vi "oax_Check DAQ Config (DSA).vi"(8 "error in (no error)":errorcluster, 10 "Tacho Type":enum16{"Analog Tacho", "Digital Tacho"}(ring), 11 "DAQ Config":T1 {"pregain" format="%.2f"; "IEPE" items=["On", "Off", "None"]; "coupling" items=["DC", "AC"]; "engineering units" items=["custom..."=0, "V"=1, "A"=21, "C"=30, "pC"=31, "s"=32, "-"=29, "Pa"=2, "N"=20, "g"=3, "m/s^2"=4, "m/s"=5, "m"=6, "mm/s"=12, "mm"=13, "micron/s"=14, "micron"=15, "in/s^2"=7, "in/s"=8, "in"=9, "mil/s"=10, "mil"=11, "rad/s^2"=16, "rad/s"=17, "rad"=18, "deg/s^2"=26, "deg/s"=27, "deg"=28, "RPM"=22, "cycle/s^2"=23, "Hz"=24, "cycle"=25, "strain"=19]; "sensor sensitivity (mV/EU)" format="%.2f"; "dB reference" format="%.1e"}) -> (0 "error out":errorcluster, 2 "dup Tacho Type":enum16{"Analog Tacho", "Digital Tacho"}(ring), 3 "dup DAQ Config":T1 {"pregain" format="%.2f"; "IEPE" items=["On", "Off", "None"]; "coupling" items=["DC", "AC"]; "engineering units" items=["custom..."=0, "V"=1, "A"=21, "C"=30, "pC"=31, "s"=32, "-"=29, "Pa"=2, "N"=20, "g"=3, "m/s^2"=4, "m/s"=5, "m"=6, "mm/s"=12, "mm"=13, "micron/s"=14, "micron"=15, "in/s^2"=7, "in/s"=8, "in"=9, "mil/s"=10, "mil"=11, "rad/s^2"=16, "rad/s"=17, "rad"=18, "deg/s^2"=26, "deg/s"=27, "deg"=28, "RPM"=22, "cycle/s^2"=23, "Hz"=24, "cycle"=25, "strain"=19]; "sensor sensitivity (mV/EU)" format="%.2f"; "dB reference" format="%.1e"})   [LabVIEW 2017]
uses:
  <vilib>/addons/Sound and Vibration/Order Analysis/Example Support/sub VIs/OAXML_DSA DAQ Config.ctl
  <vilib>/addons/_NISVFA/_Shared subVIs/Controls/svc_Engineering Units Text Ring.ctl
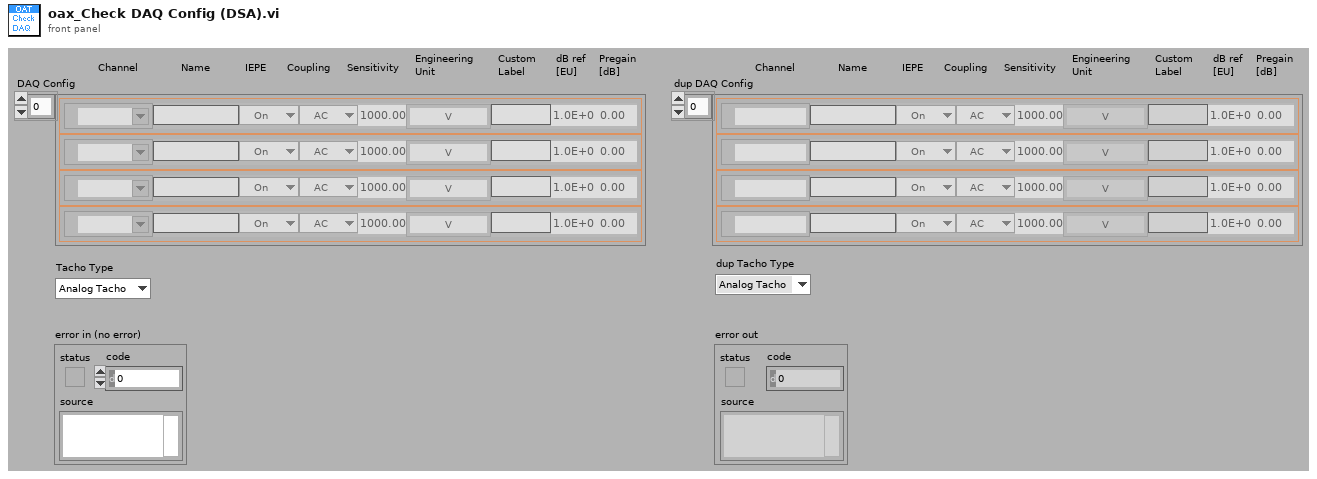
[diagram p1: front panel]
types:
  T1 = typedef "OAXML_DSA DAQ Config.ctl" = cluster{"name":string, "channel":tag, "coupling":u16, "dB reference":sgl, "sensor sensitivity (mV/EU)":dbl, "engineering units":T2, "IEPE":u16, "custom label":string, "pregain":sgl}[]
  T2 = typedef "svc_Engineering Units Text Ring.ctl" = u16
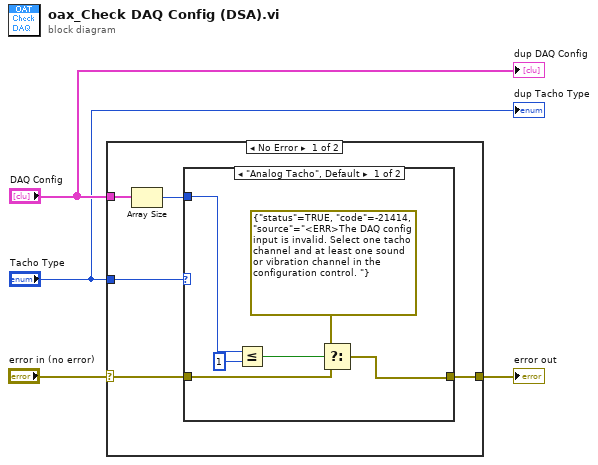
[diagram p0: block diagram]
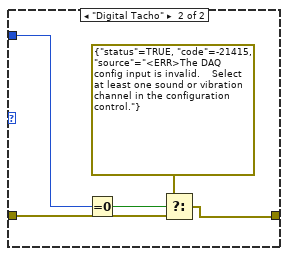
[diagram p2: hidden frame]
diagram:
  n1 = case shown="No Error" "error in (no error)" {
    selector: "error in (no error)" -> [w6 w21]
    tunnel: "DAQ Config" -> [w9 _]
    tunnel: "Tacho Type" -> [w8 _]
    tunnel: [w5 w21] -> w1
    frame No Error {
      n2 = Array Size(array=w9) -> (size(s)=w7:i32)
      n3 = case shown="\"Analog Tacho\", Default" w8 {
        tunnel: w7 -> [w12 w20]
        tunnel: w6 -> [w14 w18]
        tunnel: [w13 w16] -> w5
        frame "Analog Tacho", Default {
          n4 = Less Or Equal?(x=w12, y=1) -> (x <= y?=w15:bool)
          n5 = Select(t=errorcluster {"status"=TRUE, "code"=-21414, "source"="<ERR>The DAQ config input is invalid. Select one tacho channel and at least one sound or vibration channel in the configuration control. "}, s=w15, f=w14) -> (s? t:f=w13:errorcluster)
        }
        frame "Digital Tacho" {
          n6 = Equal To 0?(x=w20) -> (x = 0?=w17:bool)
          n7 = Select(t=errorcluster {"status"=TRUE, "code"=-21415, "source"="<ERR>The DAQ config input is invalid.    Select at least one sound or vibration channel in the configuration control."}, s=w17, f=w18) -> (s? t:f=w16:errorcluster)
        }
      }
    }
    frame Error {
    }
  }
  "error out" <- w1
  "dup DAQ Config" <- "DAQ Config"
  "dup Tacho Type" <- "Tacho Type"
